vi "Auto Calibrate.vi"(8 "error in (no error)":errorcluster, 11 "PXIe5105 in":refnum<class "PXIe5105.lvclass">) -> (0 "error out":errorcluster, 2 "Cal Passed ? (T:Yes)":bool, 3 "PXIe5105 out":refnum<class "PXIe5105.lvclass">)   [LabVIEW 2018, in "PXIe5105.lvlib" / "PXIe5105.lvclass"]
doc: "This Override method is used to call the Auto-Calibrate function of the Oscope instrument. The boolean output 'Cal Passed? (T:Yes)' carries out the auto-calibration result."
uses:
  PXIe5105.lvclass
  <instrlib>/niScope/Controls/niScope self cal option.ctl
  PXIe5105.lvclass/PXIe5105.ctl
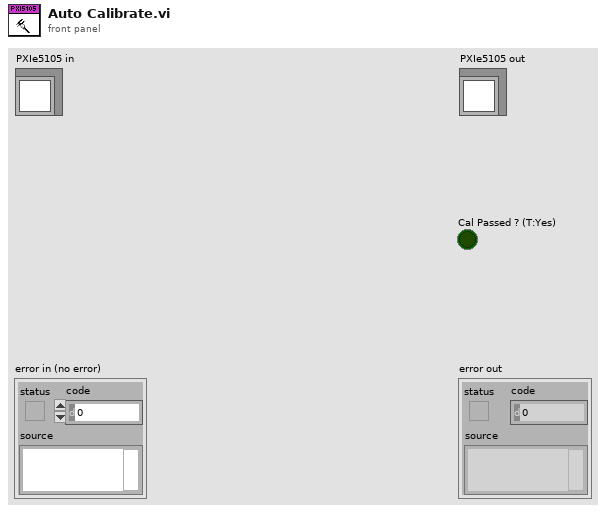
[diagram p1: front panel]
types:
  T1 = typedef "niScope self cal option.ctl" = i32
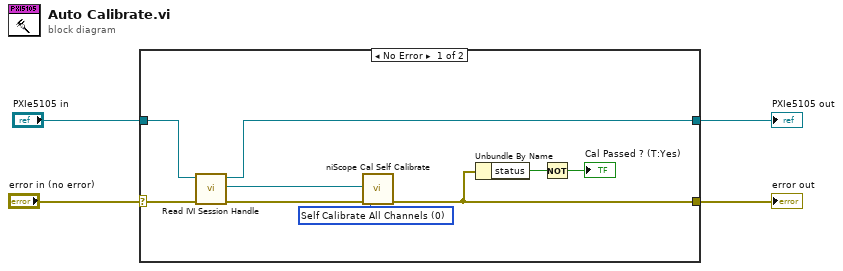
[diagram p0: block diagram]
diagram:
  n1 = case shown="No Error" "error in (no error)" {
    selector: "error in (no error)" -> [w7 w15]
    tunnel: [w12 w15] -> w3
    tunnel: [w8 w14] -> w2
    tunnel: "PXIe5105 in" -> [w9 w14]
    frame No Error {
      w13 = T1 0 items=["Self Calibrate All Channels", "Restore External Calibration"] ("Option")
      n2 = call "Read IVI Session Handle.vi"("error in (no error)"=w7, "PXIe5105 in"=w9) -> ("error out"=w6:errorcluster, "IVI Session Handle"=w5:refnum<k15>, "PXIe5105 out"=w8:refnum<class "PXIe5105.lvclass">)  [unwired: 7 in]
      n3 = call <instrlib>:"niScope Cal Self Calibrate.vi"("instrument handle"=w5, "Option"=w13, "error in"=w6) -> ("error out"=w12:errorcluster)  [unwired: 11 in, 1 out]
      n4 = Unbundle By Name(w12) -> ("status"=w11:bool)
      n5 = Not(x=w11) -> (.not. x?=→"Cal Passed ? (T:Yes)":bool)
    }
    frame Error {
    }
  }
  "error out" <- w3
  "PXIe5105 out" <- w2
